vi "AIM 664 test Import Not Parsable Configuration File.vi"(8 "error in (no error)":errorcluster, 11 "TestCase in":refnum<class "AIM 664 Import.lvclass">) -> (0 "error out":errorcluster, 3 "TestCase out":refnum<class "AIM 664 Import.lvclass">)   [LabVIEW 2020, in "AIM 664 Import.lvclass"]
uses:
  AIM 664 Import.lvclass
  <vilib>/addons/_JKI Toolkits/VI Tester/TestCase.llb/TestCase.lvclass
  <vilib>/NI/VeriStand Custom Device Testing Tools/VeriStandTestUtilities/VeriStandTestUtilities.lvlib
  Import/AIM ARINC 664 Import.lvlib
  C:/Program Files (x86)/National Instruments/LabVIEW 2020/vi.lib/addons/_JKI Toolkits/VI Tester/TestCase.llb/TestCase.lvclass
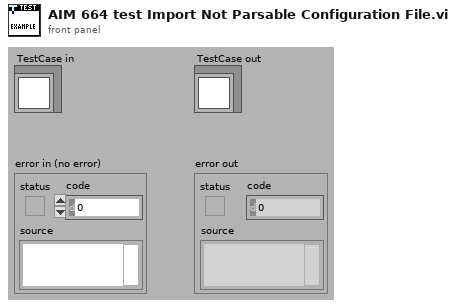
[diagram p1: front panel]
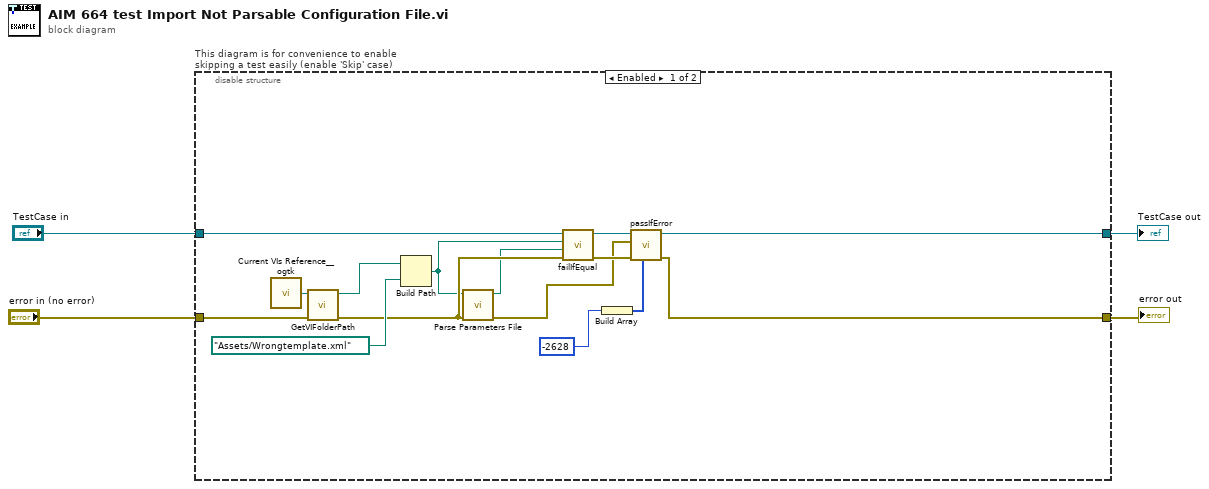
[diagram p0: block diagram]
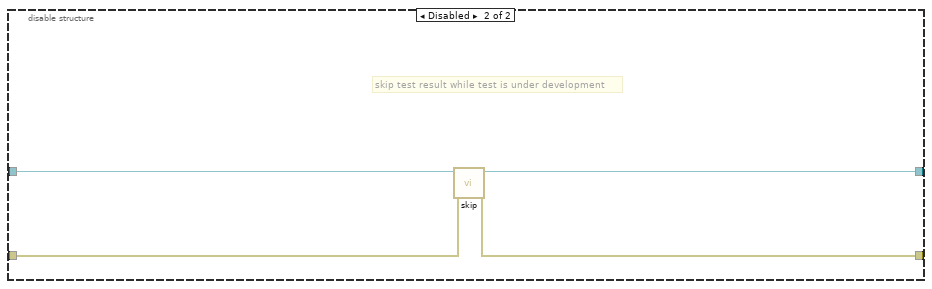
[diagram p2: hidden frame]
diagram:
  n1 = disable-structure "This diagram is for convenience to enable skipping a test easily (enable 'Skip' case)" shown="Enabled" {
    disable-tunnel: "TestCase in" -> [w11 w23]
    disable-tunnel: [w7 w21] -> w1
    disable-tunnel: [w8 w22] -> w3
    disable-tunnel: "error in (no error)" -> [w17 w20]
    frame Enabled {
      n2 = call <userlib>:"Current VIs Reference__ogtk.vi"() -> ("Current VI's reference"=w19:refnum<vi>)  [unwired: 5 in]
      n3 = call <vilib>:"GetVIFolderPath.vi"("error in (no error)"=w17, "VI Reference in"=w19) -> ("error out"=w10:errorcluster, "VI Folder Path out"=w18:path)  [unwired: 8 in]
      n4 = Build Path(base path=w18, name or relative path=path "Assets/Wrongtemplate.xml") -> (appended path=w5:path)
      n5 = call "Parse Parameters File.vi"("error in"=w10, "path to XML document"=w5) -> ("error out"=w9:errorcluster, "path to XML document out"=w6:path)  [unwired: 7 in, 1 out]
      n6 = call-dynamic "failIfEqual.vi"("error in (no error)"=w10, "y"=w6, "x"=w5, "TestCase in"=w11) -> ("error out"=w13:errorcluster, "TestCase out"=w12:refnum<class "AIM 664 Import.lvclass">)  [unwired: 6 in]
      n7 = Build Array(-2628 ("code")) -> (w15:i32[])
      n8 = call-dynamic "passIfError.vi"("passing error codes (default = any error code)"=w15, "error in (no error)"=w13, "error"=w9, "TestCase in"=w12) -> ("error out"=w8:errorcluster, "TestCase out"=w7:refnum<class "AIM 664 Import.lvclass">)  [unwired: 6 in]
    }
    frame Disabled {
      # "skip test result while test is under development"
      n9 = call <vilib>:"skip.vi"("error in (no error)"=w20, "TestCase in"=w23) -> ("error out"=w22:errorcluster, "TestCase out"=w21:refnum<class "AIM 664 Import.lvclass">)  [unwired: 8 in]
    }
  }
  "error out" <- w3
  "TestCase out" <- w1
